vi "Aerotech Acq FGV.vi"(8 "error in (no error)":errorcluster, 10 "Function":T1, 11 "Aerotech Acq Data":T2) -> (0 "error out":errorcluster, 3 "Aerotech Acq Data":T2)   [LabVIEW 2020]
uses:
  Aerotech Acq FGV Control.ctl
  Aerotech Acq FGV Function.ctl
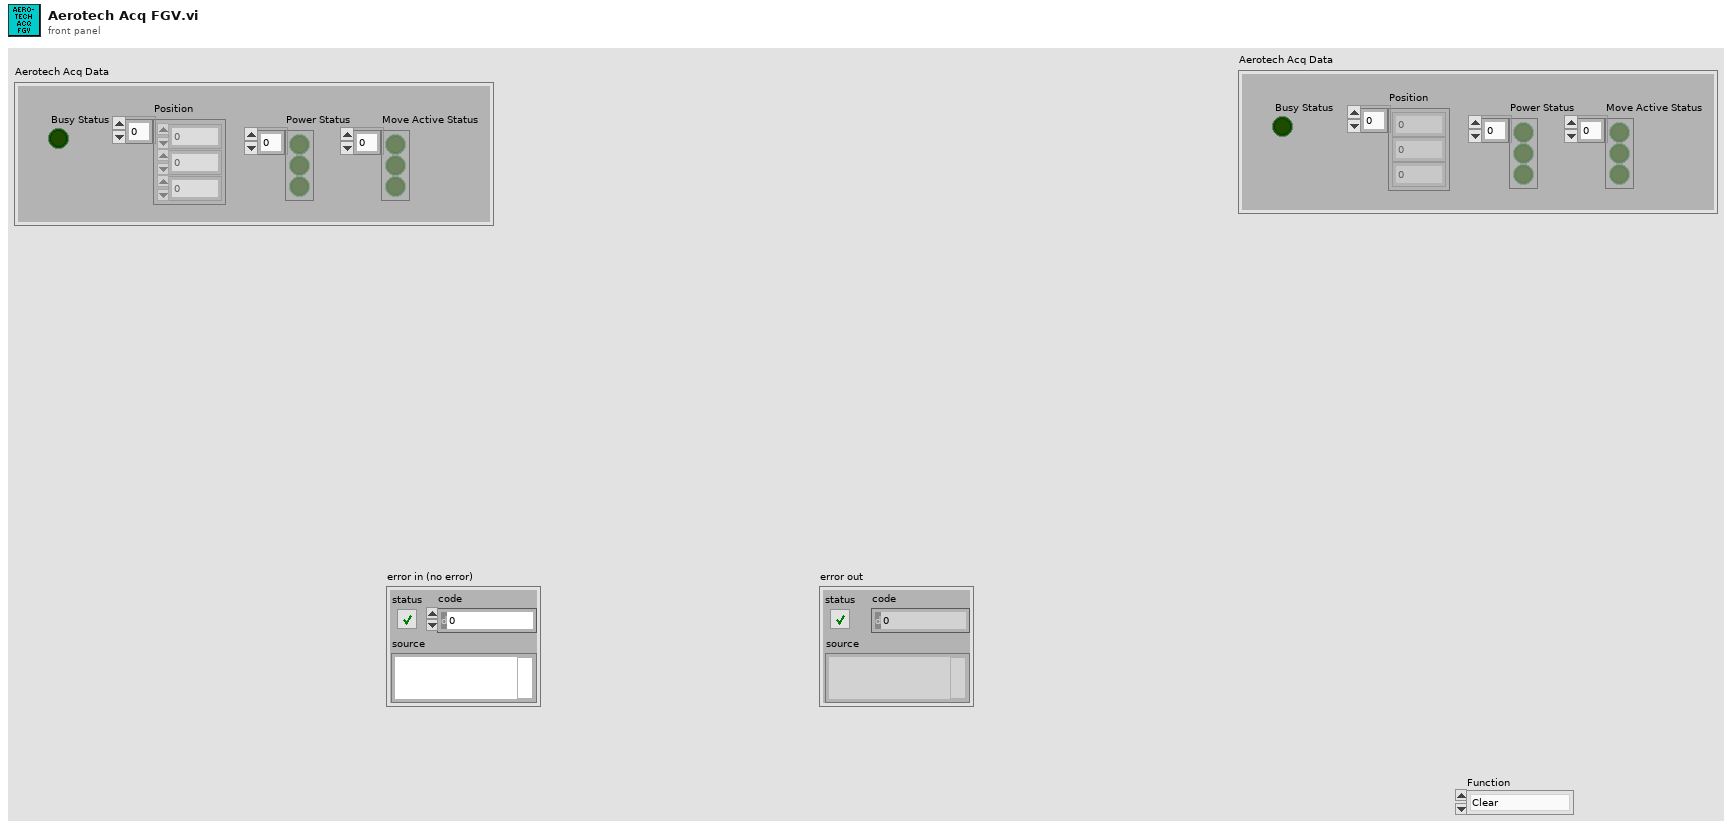
[diagram p1: front panel]
types:
  T1 = typedef "Aerotech Acq FGV Function.ctl" = enum16{"Clear", "Write", "Read"}
  T2 = typedef "Aerotech Acq FGV Control.ctl" = cluster{"Position":dbl[], "Power Status":bool[], "Move Active Status":bool[], "Busy Status":bool}
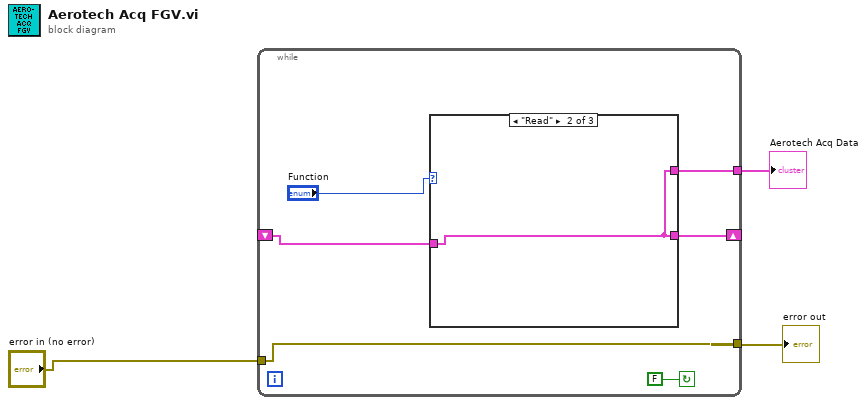
[diagram p0: block diagram]
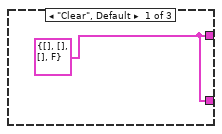
[diagram p2: hidden frame]
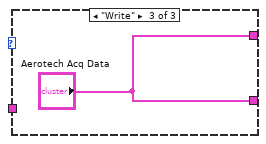
[diagram p3: hidden frame]
diagram:
  n1 = while {
    tunnel: "error in (no error)" -> [w8]
    tunnel: [w8] -> w2
    shift-right: [w6] -> _
    shift-left: _ -> [w4]
    tunnel: [w5] -> w1
    stop <- FALSE continue-if-true
    n2 = case shown="\"Read\"" "Function" {
      tunnel: [w10 w11 "Aerotech Acq Data"] -> w6
      tunnel: [w10 w11 "Aerotech Acq Data"] -> w5
      tunnel: w4 -> [_ w11 _]
      frame "Clear", Default {
        w10 = T2 {"Position"=[], "Power Status"=[], "Move Active Status"=[], "Busy Status"=FALSE} ("Aerotech Acq Data")
      }
      frame "Read" {
      }
      frame "Write" {
      }
    }
  }
  "Aerotech Acq Data" <- w1
  "error out" <- w2
